vi "jMsg_StoreNameUpdate - Rx Read.vi"(8 "error in (no error)":errorcluster, 11 "jModule":refnum<class "jModule.lvclass">) -> (0 "error out":errorcluster, 2 "Name":string, 3 "jModule":refnum<class "jModule.lvclass">, 7 "jMsg_StoreNameUpdate":refnum<class "jMsg_StoreNameUpdate.lvclass">)   [LabVIEW 2020, in "jMsg_StoreNameUpdate.lvclass"]
doc: "This VI is used to read data from the jMsg\n\n\nJSMA Message Wizard 0.2.0.5\nRob Humfeld - Jet Engineering\nCopyright (c) 2020, Jet Engineering"
uses:
  jMsg_StoreNameUpdate.lvclass
  <userlib>/JET Engineering/JSMA/Libraries/jModule Class/jModule.lvclass
  <userlib>/JET Engineering/JSMA/Libraries/jModule Class/jModule.lvclass/jModule.ctl
  jMsg_StoreNameUpdate.lvclass/jMsg_StoreNameUpdate.ctl
panel:
  in  "jMsg_StoreNameUpdate":refnum<class "jMsg_StoreNameUpdate.lvclass">
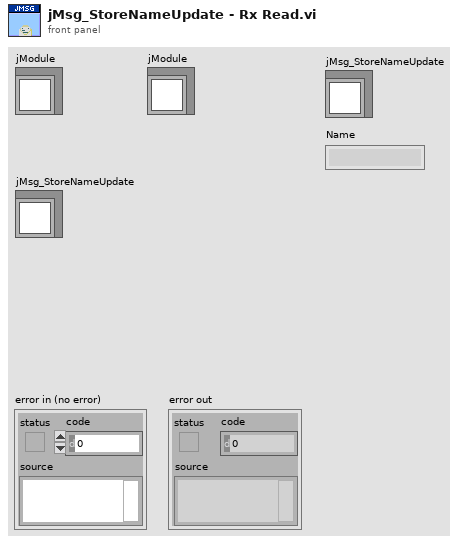
[diagram p1: front panel]
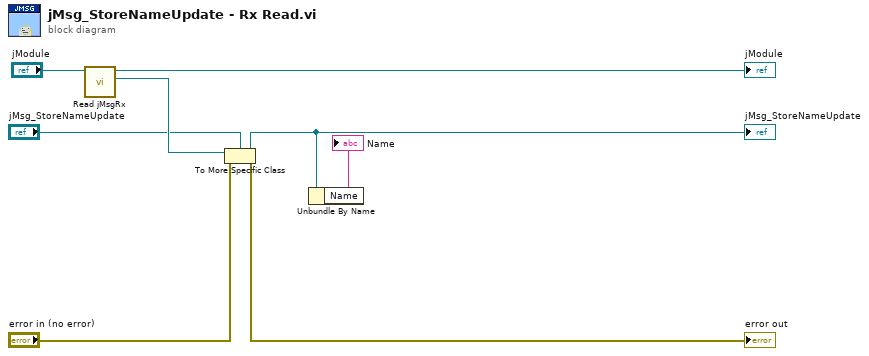
[diagram p0: block diagram]
diagram:
  n1 = call <userlib>:"Read jMsgRx.vi"("jModule in"="jModule") -> ("Received jMsg"=w5:refnum<class "jMsg.lvclass">, "jModule out"=→"jModule":refnum<class "jModule.lvclass">)  [unwired: 8 in, 1 out]
  n2 = To More Specific Class(target class="jMsg_StoreNameUpdate", reference=w5, error in="error in (no error)") -> (specific class reference=w8:refnum<class "jMsg_StoreNameUpdate.lvclass">, error out=→"error out":errorcluster)
  "jMsg_StoreNameUpdate" <- w8
  n3 = Unbundle By Name(w8) -> ("Name"=→"Name":string)
